vi "Get Revisions Property Name.vi"(11 "module identifier":string) -> (3 "module revision property name":string)   [LabVIEW 2020, in "Routing and Faulting Scripting.lvlib"]
uses:
  Routing and Faulting Scripting.lvlib
  Constants/Scripting Constants.vi
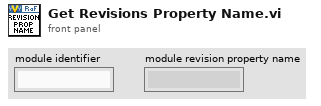
[diagram p1: front panel]
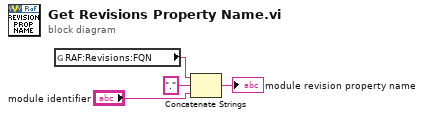
[diagram p0: block diagram]
diagram:
  n1 = global read "Scripting Constants.vi" "RAF:Revisions:FQN"() -> (w1:string)
  n2 = Concatenate Strings(w1, "." ("string"), "module identifier") -> (→"module revision property name":string)
